vi "poly_dialog_interrupt_2btn.vi"(6 "F button name (\"Cancel\")":string="Cancel", 8 "error in":errorcluster caption="Error in (no error)", 9 "T button name (\"OK\")":string="OK", 10 "message":string) -> (0 "error out":errorcluster, 2 "T button?":bool)   [LabVIEW 2015]
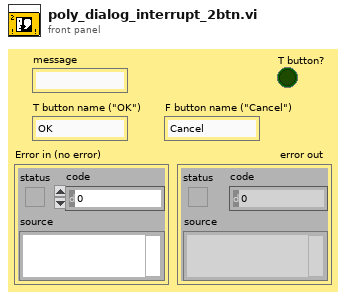
[diagram p1: front panel]
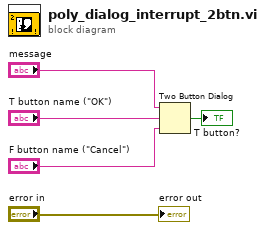
[diagram p0: block diagram]
diagram:
  n1 = Two Button Dialog(message="message", 1:"F button name (\"Cancel\")", 2:"T button name (\"OK\")") -> (T button?=→"T button?":bool)
  "error out" <- "error in"
